vi "KN-ReadVISAPamams.vi"(0 "名称或相对路径":string="UserDefine.ini", 11 "error in (no error)":errorcluster caption="错误输入（无错误）") -> (4 "VISA1 Param":string[](array[string]), 15 "error out":errorcluster caption="错误输出")   [LabVIEW 2017]
uses:
  Global System.vi
  <vilib>/Utility/config.llb/NI_LVConfig.lvlib
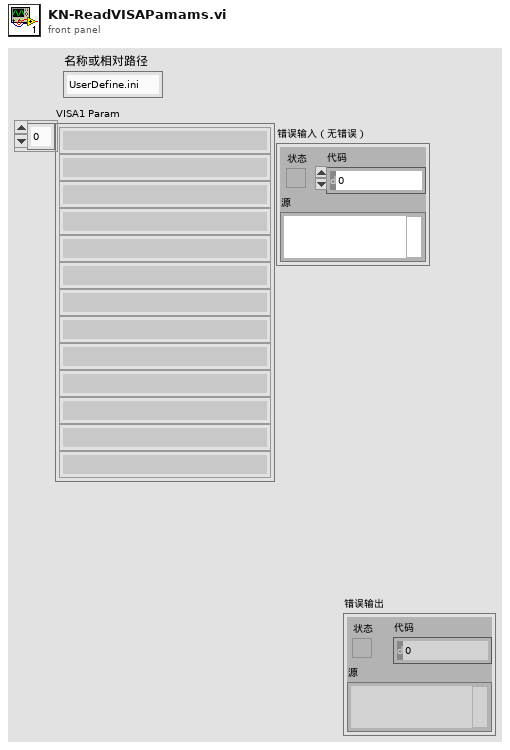
[diagram p1: front panel]
types:
  T1 = typedef "NI_LVConfig.lvlib/Config Data RefNum.ctl" = refnum<k1>
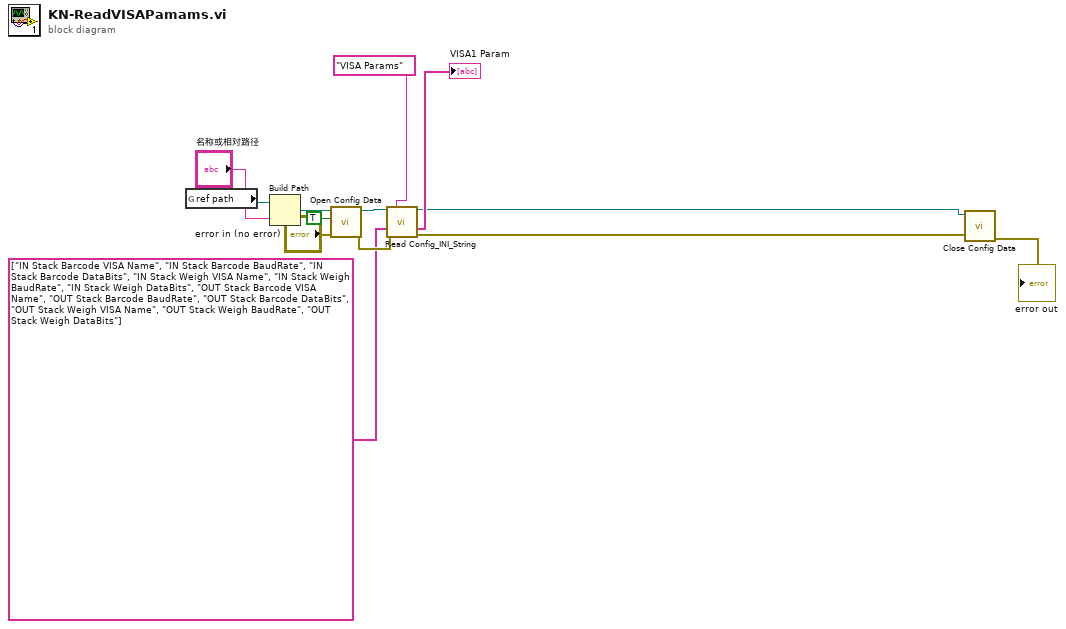
[diagram p0: block diagram]
diagram:
  n1 = global read "Global System.vi" "ref path"() -> (w7:path)
  n2 = Build Path(base path=w7, name or relative path="名称或相对路径") -> (appended path=w10:path)
  n3 = call <vilib>:"Open Config Data.vi"("error in (no error)"="error in (no error)", "create file if necessary (T)"=TRUE, "configuration file path"=w10) -> ("error out"=w12:errorcluster, "refnum"=w11:T1)  [unwired: 6 in, 1 out]
  n4 = call "Read Config_INI_String.vi"("refnum"=w11, "section"="VISA Params", "Keys"=string[] ["IN Stack Barcode VISA Name", "IN Stack Barcode BaudRate", "IN Stack Barcode DataBits", "IN Stack Weigh VISA Name", "IN Stack Weigh BaudRate", "IN Stack Weigh DataBits", "OUT Stack Barcode VISA Name", "OUT Stack Barcode BaudRate", "OUT Stack Barcode DataBits", "OUT Stack Weigh VISA Name", "OUT Stack Weigh BaudRate", "OUT Stack Weigh DataBits"], "error in (no error)"=w12) -> ("refnum out"=w2:T1, "Outputs"=→"VISA1 Param":string[], "error out"=w1:errorcluster)  [unwired: 9 in]
  n5 = call <vilib>:"Close Config Data.vi"("error in (no error)"=w1, "refnum"=w2) -> ("error out"=→"error out":errorcluster)  [unwired: 8 in, 1 out]
